vi "Read ADU Packet.vi"(8 "error in":errorcluster, 10 "isMaster (f)":bool, 11 "ASCII transmission data unit in":refnum<class "ASCII Data Unit.lvclass">) -> (0 "error out":errorcluster, 1 "modbus data unit":refnum<class "Modbus Data Unit.lvclass">, 3 "ASCII transmission data unit out":refnum<class "ASCII Data Unit.lvclass">, 5 "PDU Valid?":bool)   [LabVIEW 2021, in "ASCII Data Unit.lvclass"]
uses:
  ASCII Data Unit.lvclass
  D:/my_projects/projects/Algorithms/Labview/21/Modbus_v121c/Transmission Data Unit/Transmission Data Unit.lvclass
  D:/my_projects/projects/Algorithms/Labview/21/Modbus_v121c/Transmission Data Unit/Serial Interface/Serial Data Unit.lvclass
  Modbus Data Unit/Modbus Data Unit.lvclass
  Serial Interface/Serial Data Unit.lvclass/Serial Data Unit.ctl
  Transmission Data Unit.lvclass/Transmission Data Unit.ctl
  ASCII Data Unit.lvclass/ASCII Data Unit.ctl
  Serial Interface/Serial acquisition states.ctl
  Modbus Data Unit/Modbus Data Unit.lvclass/Modbus Data Unit.ctl
  <vilib>/ErrorRing/Error Ring.xnode
  Transmission Data Unit.lvclass
  Serial Interface/Serial Data Unit.lvclass
  Network Interface/Serial Interface/Serial Shared Components/Serial Shared Components.lvlib
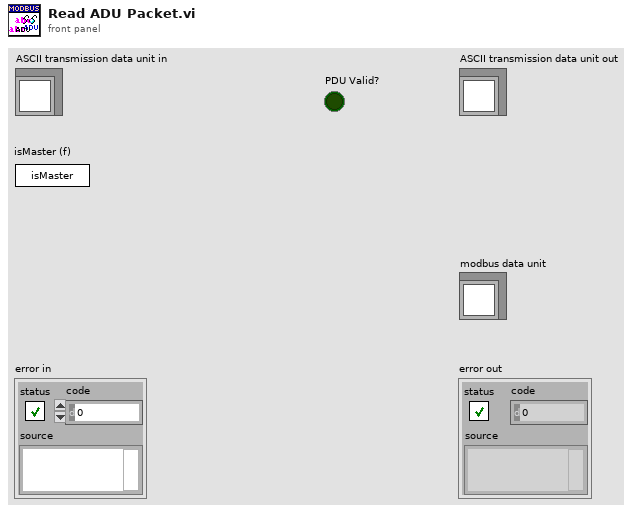
[diagram p1: front panel]
types:
  T1 = typedef "Serial Data Unit.lvclass/Serial acquisition states.ctl" = enum16{"Wait for frame", "Check for validity"}
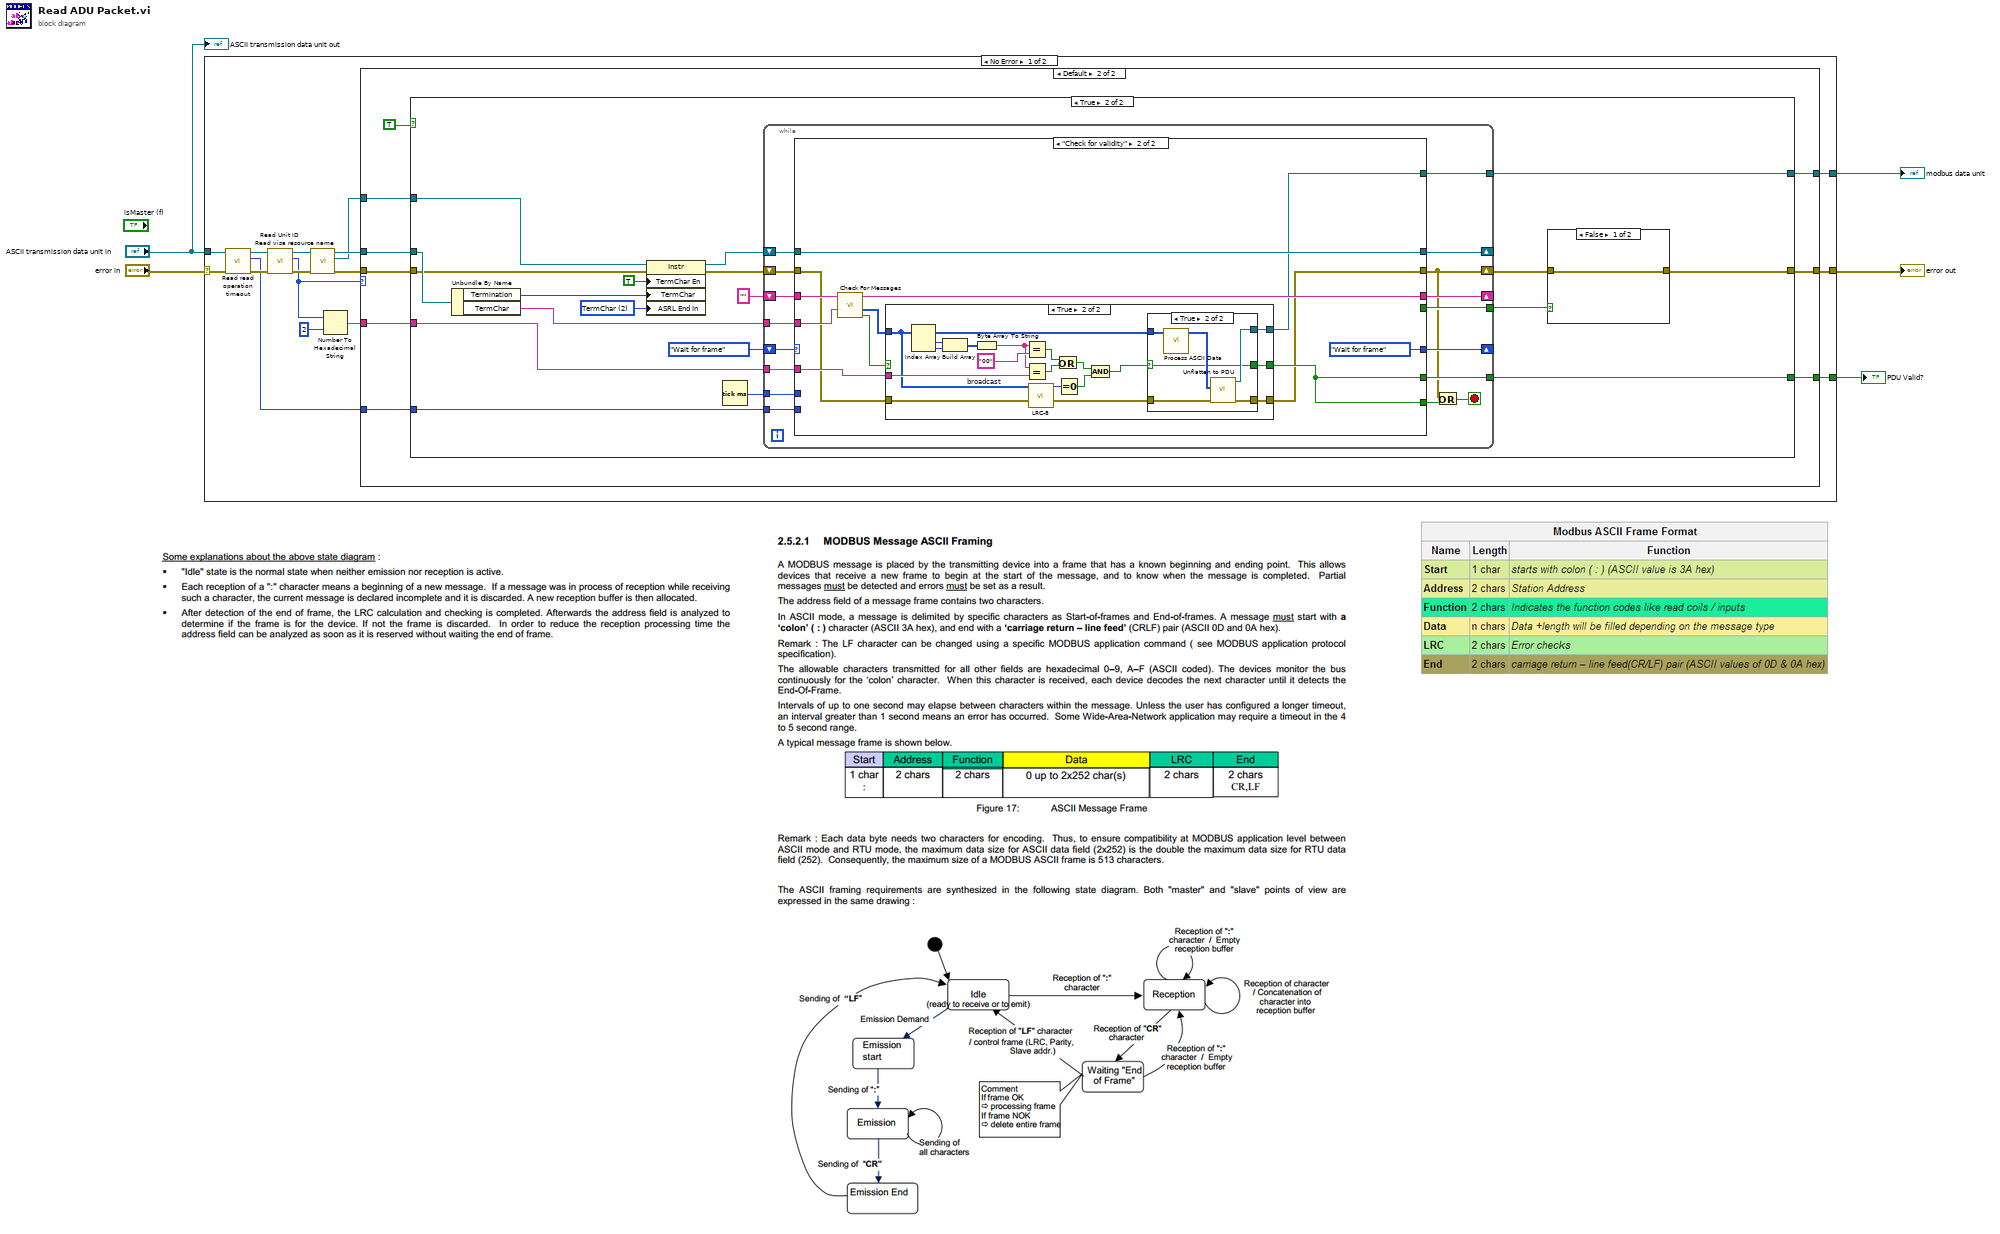
[diagram p0: block diagram]
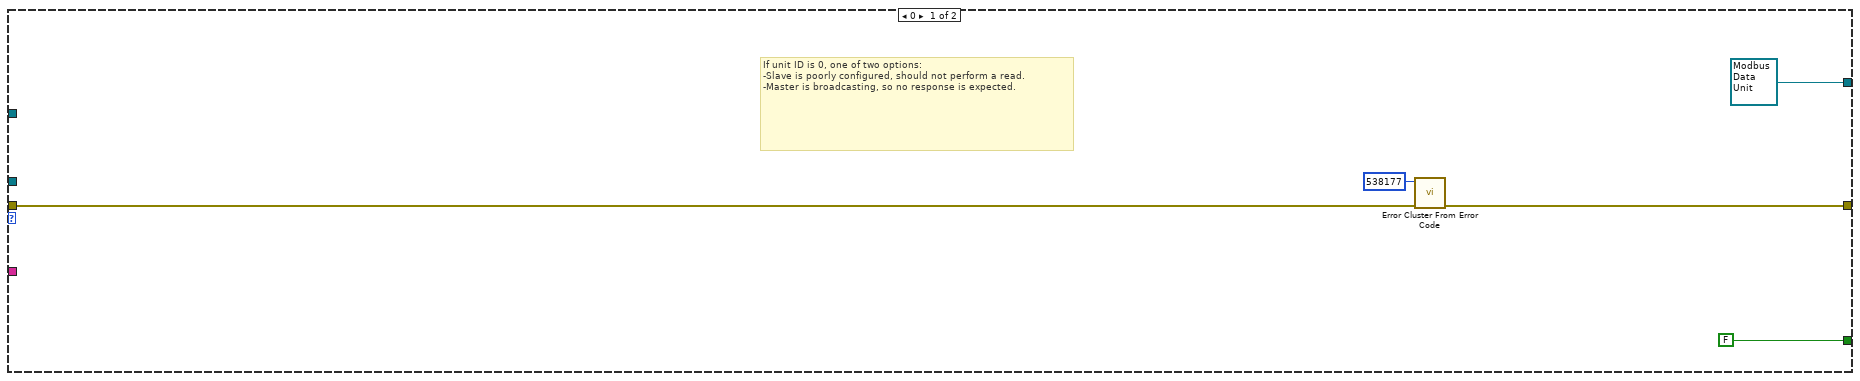
[diagram p2: hidden frame]
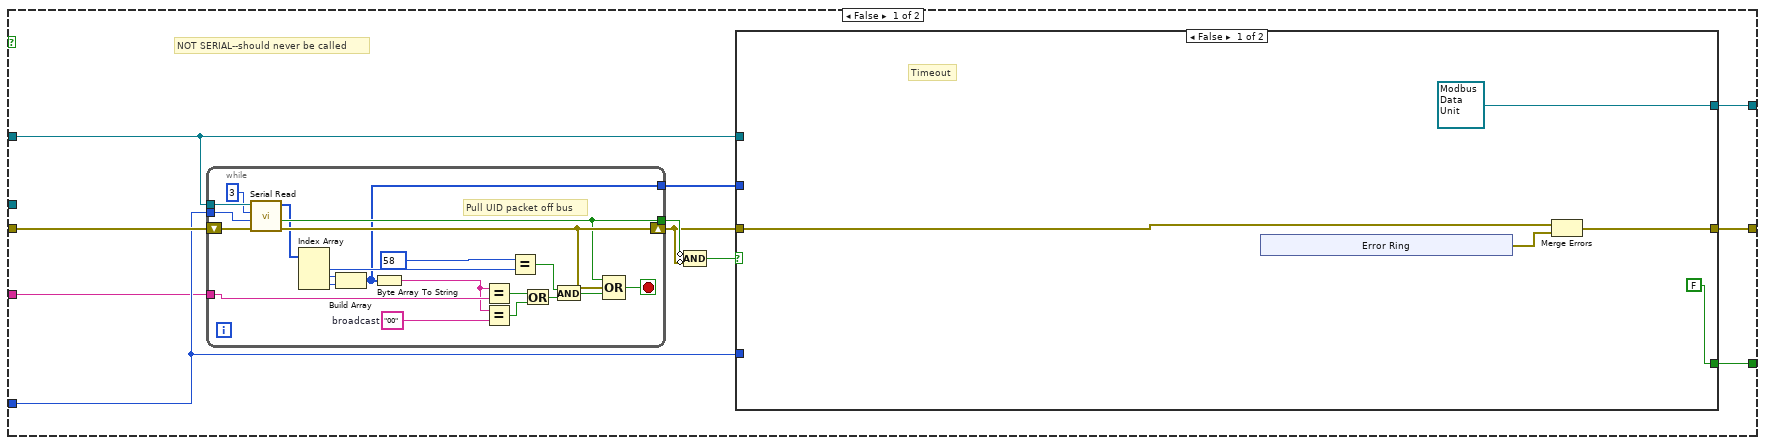
[diagram p3: hidden frame]
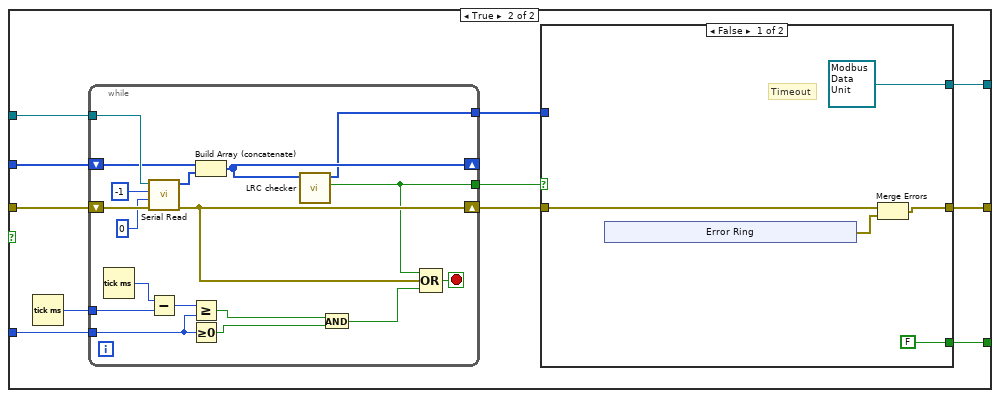
[diagram p4: hidden frame]
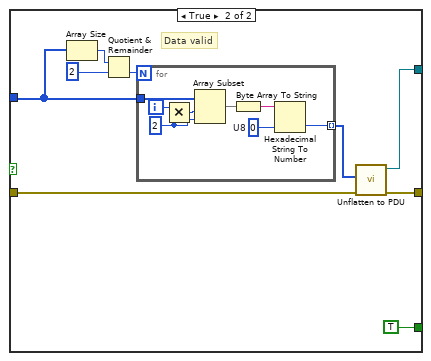
[diagram p5: hidden frame]
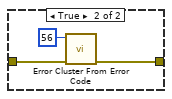
[diagram p6: hidden frame]
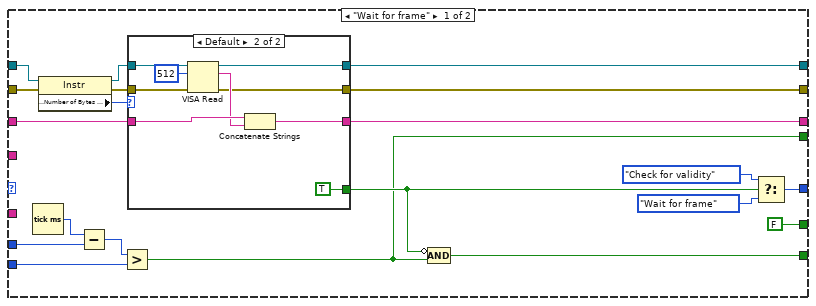
[diagram p7: hidden frame]
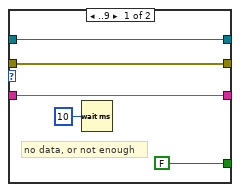
[diagram p8: hidden frame]
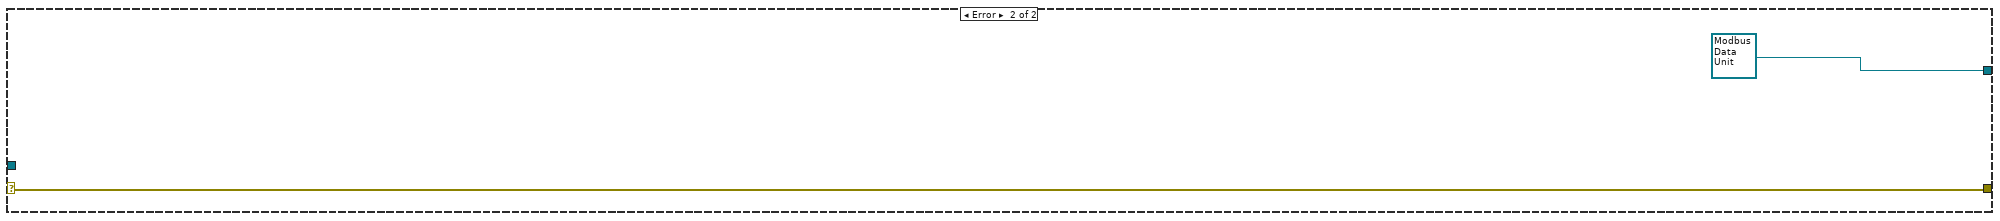
[diagram p11: hidden frame]
diagram:
  n1 = case shown="No Error" "error in" {
    selector: "error in" -> [w13 w246]
    tunnel: [w21 w246] -> w4
    tunnel: "ASCII transmission data unit in" -> [w14 _]
    tunnel: [w20 refnum<class "Modbus Data Unit.lvclass"> refnum ("modbus data unit")] -> w5
    tunnel: [w19 _] -> w3
    frame No Error {
      n2 = call "Read read operation timeout.vi"("error in (no error)"=w13, "transmission data unit in"=w14) -> ("error out"=w16:errorcluster, "read operation timeout"=w7:i32, "transmission data unit out"=w15:refnum<class "ASCII Data Unit.lvclass">)  [unwired: 7 in]
      n3 = call "Read Unit ID.vi"("error in"=w16, "transmission data unit in"=w15) -> ("error out"=w11:errorcluster, "unit ID"=w10:u8, "transmission data unit out"=w12:refnum<class "ASCII Data Unit.lvclass">)  [unwired: 7 in]
      n4 = call "Read visa resource name.vi"("error in (no error)"=w11, "Serial Data Unit in"=w12) -> ("error out"=w8:errorcluster, "visa resource name"=w6:refnum<visa-resource-name>, "Serial Data Unit out"=w9:refnum<class "ASCII Data Unit.lvclass">)  [unwired: 7 in]
      n5 = Number To Hexadecimal String(1:i16 2 ("width (-)"), 2:w10) -> (0:w17:string)
      n6 = case shown="Default" w10 {
        tunnel: w8 -> [w26 w31]
        tunnel: [w23 w35] -> w21
        tunnel: [refnum<class "Modbus Data Unit.lvclass"> refnum ("modbus data unit out") w34] -> w20
        tunnel: w6 -> [_ w30]
        tunnel: w7 -> [_ w33]
        tunnel: [FALSE w32] -> w19
        tunnel: w17 -> [_ w29]
        tunnel: w9 -> [_ w28]
        frame 0 {
          # "If unit ID is 0, one of two options:\n-Slave is poorly configured, should not perform a read.\n-Master is broadcasting, so no response is expected."
          n7 = call <vilib>:"Error Cluster From Error Code.vi"("error in (no error)"=w26, "error code (0)"=538177) -> ("error out"=w23:errorcluster)  [unwired: 7 in]
        }
        frame Default {
          n8 = case shown="True" TRUE {
            tunnel: w31 -> [w46 w140]
            tunnel: [w42 w134] -> w35
            tunnel: [w41 w133] -> w34
            tunnel: w30 -> [w40 w132]
            tunnel: w33 -> [w38 w141]
            tunnel: [w37 w139] -> w32
            tunnel: w29 -> [w36 w137]
            tunnel: w28 -> [_ w148]
            frame False {
              # "NOT SERIAL--should never be called"
              n9 = while {
                shift-right: [w128] -> w43
                shift-left: w46 -> [w131]
                tunnel: w38 -> [w126]
                tunnel: [w124] -> w45
                tunnel: [w116] -> w39
                tunnel: w40 -> [w130]
                tunnel: w36 -> [w117]
                stop <- w129 stop-if-true
                w111 = "00"  # broadcast
                # "Pull UID packet off bus"
                n10 = call "Serial Read.vi"("error in"=w131, "timeout (ms)"=w126, "bytes to read"=3, "Visa Resource"=w130) -> ("error out"=w128:errorcluster, "timed out?"=w124:bool, "data"=w123:u8[])  [unwired: 5 in]
                n11 = Index Array(array=w123) -> (element #1=w121:u8, element #2=w119:u8, element #3=w118:u8)  [unwired: 3 in]
                n12 = Build Array(w119, w118) -> (w116:u8[])
                n13 = Byte Array To String(unsigned byte array=w116) -> (string=w112:string)
                n14 = Equal?(x=w112, y=w117) -> (x = y?=w114:bool)
                n15 = Equal?(x=w112, y=w111) -> (x = y?=w113:bool)
                n16 = Equal?(x=u8 58 ("y"), y=w121) -> (x = y?=w120:bool)
                n17 = Or(x=w114, y=w113) -> (x .or. y?=w115:bool)
                n18 = And(x=w120, y=w115) -> (x .and. y?=w125:bool)
                n19 = Compound Arithmetic op=OR(w124, w128, w125) -> (w129:bool)
              }
              n20 = Compound Arithmetic op=AND(invert w45, invert w43) -> (w44:bool)
              n21 = case shown="False" w44 {
                tunnel: w43 -> [w49 w66]
                tunnel: [w50 w58] -> w42
                tunnel: [refnum<class "Modbus Data Unit.lvclass"> refnum ("modbus data unit out") w59] -> w41
                tunnel: w40 -> [_ w62]
                tunnel: w39 -> [_ w63]
                tunnel: w38 -> [_ w64]
                tunnel: [FALSE w56] -> w37
                frame False {
                  # "Timeout"
                  n22 = xnode "Error Ring"() -> ("error out"=w51:errorcluster)
                  n23 = Merge Errors(w49, w51) -> (w50:errorcluster)
                }
                frame True {
                  n24 = Tick Count (ms)() -> (millisecond timer value=w65:u32)
                  n25 = while {
                    shift-right: [w96] -> w60
                    shift-left: w66 -> [w102]
                    tunnel: w65 -> [w110]
                    tunnel: w64 -> [w107]
                    shift-right: [w95] -> _
                    shift-left: w63 -> [w98]
                    tunnel: w62 -> [w101]
                    tunnel: [w93] -> w61
                    tunnel: [w94] -> w57
                    stop <- w104 stop-if-true
                    n26 = Tick Count (ms)() -> (millisecond timer value=w109:u32)
                    n27 = call "Serial Read.vi"("error in"=w102, "timeout (ms)"=0 ("timeout"), "bytes to read"=-1, "Visa Resource"=w101) -> ("error out"=w96:errorcluster, "data"=w97:u8[])  [unwired: 5 in, 1 out]
                    n28 = Subtract(x=w109, y=w110) -> (x-y=w108:u32)
                    n29 = Greater Or Equal?(x=w108, y=w107) -> (x >= y?=w105:bool)
                    n30 = Greater Or Equal To 0?(x=w107) -> (x >= 0?=w106:bool)
                    n31 = Build Array (concatenate)(w98, w97) -> (w95:u8[])
                    n32 = call "LRC checker.vi"("Data In"=w95) -> ("Valid?"=w93:bool, "Function Data Out"=w94:u8[])  [unwired: 9 in]
                    n33 = And(x=w105, y=w106) -> (x .and. y?=w103:bool)
                    n34 = Compound Arithmetic op=OR(w93, w96, w103) -> (w104:bool)
                  }
                  n35 = case shown="False" w61 {
                    tunnel: w60 -> [w69 w82]
                    tunnel: [refnum<class "Modbus Data Unit.lvclass"> refnum ("modbus data unit") w83] -> w59
                    tunnel: [w68 w84] -> w58
                    tunnel: w57 -> [_ w77]
                    tunnel: [FALSE TRUE] -> w56
                    frame False {
                      # "Timeout"
                      n36 = xnode "Error Ring"() -> ("error out"=w70:errorcluster)
                      n37 = Merge Errors(w69, w70) -> (w68:errorcluster)
                    }
                    frame True {
                      # "Data valid"
                      n38 = Array Size(array=w77) -> (size(s)=w81:i32)
                      n39 = Quotient & Remainder(x=w81, y=2) -> (floor(x/y)=w79:i32)  [unwired: 1 out]
                      n40 = for {
                        N: w79 -> [_]
                        tunnel: w77 -> [w92]
                        tunnel: [w85] -> w78 mode=indexing
                        i -> [w91]
                        w86 = u8 0  # U8
                        w90 = 2 ("length")
                        n41 = Multiply(x=w91, y=w90) -> (x*y=w89:i32)
                        n42 = Array Subset(array=w92, index=w89, length=w90) -> (w88:u8[])
                        n43 = Byte Array To String(unsigned byte array=w88) -> (string=w87:string)
                        n44 = Hexadecimal String To Number(string=w87, default (0uL)=w86) -> (number=w85:u8)  [unwired: 2 out]
                      }
                      n45 = call "Unflatten to PDU.vi"("error in"=w82, "modbus data unit data"=w78) -> ("error out"=w84:errorcluster, "modbus data unit out"=w83:refnum<class "Modbus Data Unit.lvclass">)  [unwired: 8 in]
                    }
                  }
                }
              }
            }
            frame True {
              w149 = u16 2 items=["None", "Last Bit", "TermChar"] ("Serial Settings:End Mode for Reads")
              n46 = Unbundle By Name(w148) -> ("Termination"=w147:u8, "TermChar"=w138:string)
              n47 = property class="Instr"(reference=w132, error in=w140, "TermChar En"=TRUE ("Message Based Settings:Termination Character Enable"), "TermChar"=w147, "ASRL End In"=w149) -> (reference out=w145:refnum<visa-resource-name>, error out=w144:errorcluster)
              n48 = Tick Count (ms)() -> (millisecond timer value=w142:u32)
              n49 = while {
                shift-right: [w170] -> _
                shift-left: Serial_acquisition_states."Wait for frame" ("Serial Acquisition States") -> [w171]
                shift-right: [w155] -> w135
                shift-left: w144 -> [w168]
                shift-right: [w162] -> _
                shift-left: w145 -> [w169]
                shift-right: [w166] -> _
                shift-left: "" -> [w167]
                tunnel: w142 -> [w165]
                tunnel: w141 -> [w164]
                tunnel: [w161] -> w139
                tunnel: w138 -> [w160]
                tunnel: w137 -> [w159]
                tunnel: [w158] -> w136
                tunnel: [w157] -> w133
                stop <- w156 stop-if-true
                n50 = case shown="\"Check for validity\"" w171 {
                  tunnel: [w191 Serial_acquisition_states."Wait for frame" ("Serial Acquisition States")] -> w170
                  tunnel: w169 -> [w186 w216]
                  tunnel: w168 -> [w185 w207]
                  tunnel: w167 -> [w184 w215]
                  tunnel: [w183 w213] -> w166
                  tunnel: w165 -> [w181 _]
                  tunnel: w164 -> [w179 _]
                  tunnel: [w174 w209] -> w163
                  tunnel: [w176 w206] -> w155
                  tunnel: [w175 w216] -> w162
                  tunnel: [FALSE w209] -> w161
                  tunnel: w160 -> [_ w214]
                  tunnel: w159 -> [_ w211]
                  tunnel: [w172 _] -> w158
                  tunnel: [_ w208] -> w157
                  frame "Wait for frame" {
                    n51 = Tick Count (ms)() -> (millisecond timer value=w182:u32)
                    n52 = property class="Instr"(reference=w186, error in=w185) -> (reference out=w188:refnum<visa-resource-name>, error out=w177:errorcluster, "Serial Settings:Number of Bytes at Serial Port"=w187:u32)
                    n53 = Subtract(x=w182, y=w181) -> (x-y=w180:u32)
                    n54 = Greater?(x=w180, y=w179) -> (0:w172:bool)
                    n55 = case shown="Default" w187 {
                      tunnel: w188 -> [w192 w205]
                      tunnel: w184 -> [w195 w204]
                      tunnel: [w195 w202] -> w183
                      tunnel: [FALSE TRUE] -> w178
                      tunnel: w177 -> [w193 w200]
                      tunnel: [w193 w199] -> w176
                      tunnel: [w192 w198] -> w175
                      frame ..9 {
                        # "no data, or not enough"
                        n56 = Wait (ms)(milliseconds to wait=u32 10) -> ()  [unwired: 1 out]
                      }
                      frame Default {
                        n57 = VISA Read(VISA resource name=w205, byte count=u32 512, error in (no error)=w200) -> (VISA resource name out=w198:refnum<visa-resource-name>, read buffer=w203:string, error out=w199:errorcluster)  [unwired: 1 out]
                        n58 = Concatenate Strings(w204, w203) -> (w202:string)
                      }
                    }
                    n59 = Compound Arithmetic op=AND(invert w178, w172) -> (w174:bool)
                    n60 = Select(t=Serial_acquisition_states."Check for validity" ("Serial Acquisition States"), s=w178, f=Serial_acquisition_states."Wait for frame" ("Serial Acquisition States")) -> (s? t:f=w191:T1)
                  }
                  frame "Check for validity" {
                    n61 = call "Check For Messages.vi"("Term Char"=w214, "Input String"=w215) -> ("found?"=w210:bool, "data"=w212:u8[], "Remaining String"=w213:string)  [unwired: 7 in]
                    n62 = case shown="True" w210 {
                      selector: w210 -> [w219 _]
                      tunnel: w212 -> [_ w225]
                      tunnel: w211 -> [_ w226]
                      tunnel: w207 -> [w218 w224]
                      tunnel: [w219 w220] -> w209
                      tunnel: [_ w223] -> w208
                      tunnel: [w218 w222] -> w206
                      frame False {
                      }
                      frame True {
                        w234 = "00"  # broadcast
                        n63 = Index Array(array=w225) -> (element #1=w230:u8, element #2=w231:u8)  [unwired: 2 in]
                        n64 = Build Array(w230, w231) -> (w229:u8[])
                        n65 = Byte Array To String(unsigned byte array=w229) -> (string=w233:string)
                        n66 = Equal?(x=w233, y=w234) -> (x = y?=w232:bool)
                        n67 = Equal?(x=w233, y=w226) -> (x = y?=w227:bool)
                        n68 = call "LRC-8.vi"("data"=w225) -> ("LRC-8"=w235:u8)  [unwired: 10 in]
                        n69 = Or(x=w232, y=w227) -> (x .or. y?=w228:bool)
                        n70 = Equal To 0?(x=w235) -> (x = 0?=w236:bool)
                        n71 = Compound Arithmetic op=AND(w228, w236) -> (w221:bool)
                        n72 = case shown="True" w221 {
                          selector: w221 -> [w237 w239]
                          tunnel: w225 -> [_ w244]
                          tunnel: w224 -> [w238 w243]
                          tunnel: [_ w241] -> w223
                          tunnel: [w238 w240] -> w222
                          tunnel: [w237 w239] -> w220
                          frame False {
                          }
                          frame True {
                            n73 = call "Process ASCII Data.vi"("data"=w244) -> ("pdu"=w242:u8[])  [unwired: 10 in]
                            n74 = call "Unflatten to PDU.vi"("error in"=w243, "modbus data unit data"=w242) -> ("error out"=w240:errorcluster, "modbus data unit out"=w241:refnum<class "Modbus Data Unit.lvclass">)  [unwired: 8 in]
                          }
                        }
                      }
                    }
                  }
                }
                n75 = Or(x=w155, y=w163) -> (x .or. y?=w156:bool)
              }
              n76 = case shown="False" w136 {
                tunnel: w135 -> [w151 w154]
                tunnel: [w151 w152] -> w134
                frame False {
                }
                frame True {
                  n77 = call <vilib>:"Error Cluster From Error Code.vi"("error in (no error)"=w154, "error code (0)"=56) -> ("error out"=w152:errorcluster)  [unwired: 7 in]
                }
              }
            }
          }
        }
      }
    }
    frame Error {
    }
  }
  "modbus data unit" <- w5
  "error out" <- w4
  "PDU Valid?" <- w3
  "ASCII transmission data unit out" <- "ASCII transmission data unit in"
